vi "get_software_buffer_size.vi"(8 "error in (no error)":errorcluster, 11 "GenericDAQ.lvclass in":refnum<class "GenericDAQ.lvclass">) -> (0 "error out":errorcluster, 2 "software buffer size":i32, 3 "GenericDAQ.lvclass out":refnum<class "GenericDAQ.lvclass">)   [LabVIEW 2010, in "GenericDAQ.lvclass"]
uses:
  GenericDAQ.lvclass
  GenericDAQ.lvclass/GenericDAQ.ctl
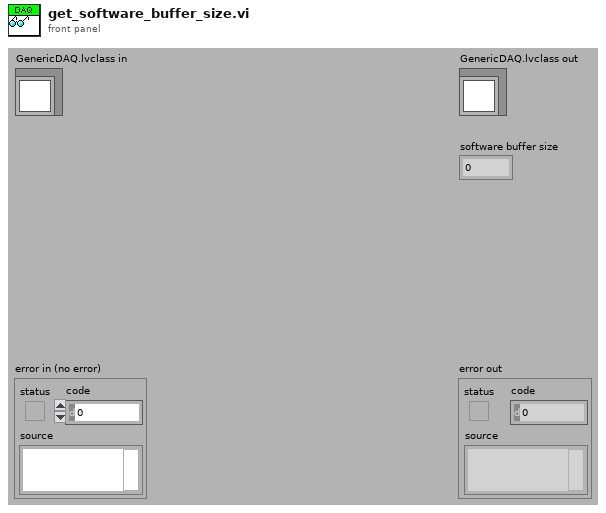
[diagram p1: front panel]
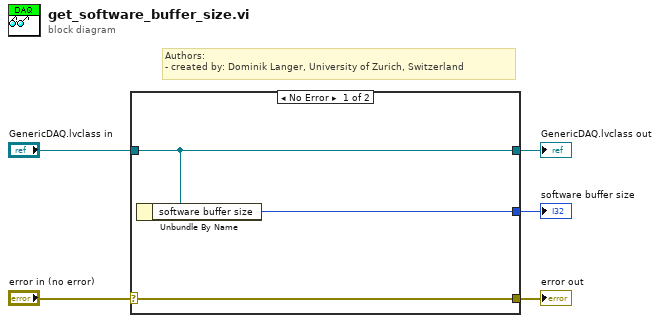
[diagram p0: block diagram]
diagram:
  # "Authors: \n- created by: Dominik Langer, University of Zurich, Switzerland"
  n1 = case shown="No Error" "error in (no error)" {
    selector: "error in (no error)" -> [w8 w9]
    tunnel: [w8 w9] -> w4
    tunnel: [w7 w10] -> w2
    tunnel: "GenericDAQ.lvclass in" -> [w7 w10]
    tunnel: [w6 _] -> w1
    frame No Error {
      n2 = Unbundle By Name(w7) -> ("software buffer size"=w6:i32)
    }
    frame Error {
    }
  }
  "error out" <- w4
  "GenericDAQ.lvclass out" <- w2
  "software buffer size" <- w1
